vi "04-ClusterEscala.vi"() -> ()   [LabVIEW 2020]
panel:
  in  "Tab Control":enum32{"Cluster"}(tab)
  out "Cluster":T1 {"Tank" scale=0.0..500.0; "Gauge" scale=0.0..500.0; "Thermometer" scale=0.0..100.0}
  in  "Cluster 2":T2
  out "x*y":cluster{dbl, dbl, dbl}
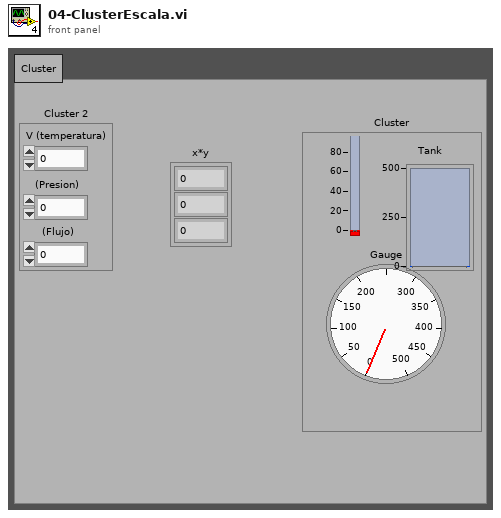
[diagram p1: front panel]
types:
  T1 = cluster{"Thermometer":dbl, "Gauge":dbl, "Tank":dbl}
  T2 = cluster{"V (temperatura)":dbl, "(Presion)":dbl, "(Flujo)":dbl}
  T3 = cluster{"°C/V":i32, "(I/seg)/V":i32, "(N/m^2)/V":i32}
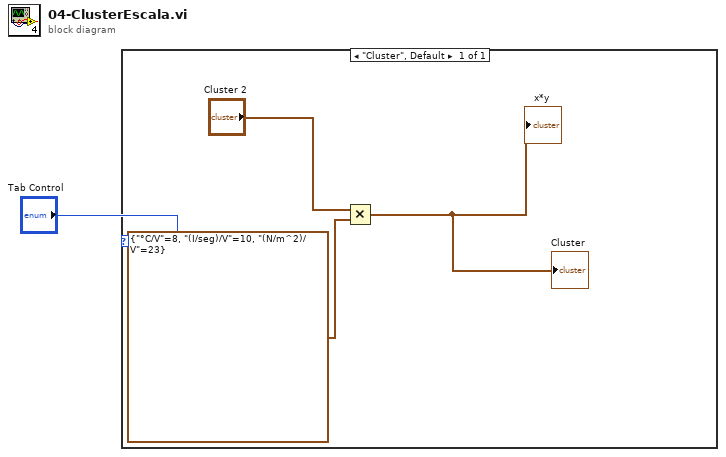
[diagram p0: block diagram]
diagram:
  n1 = case shown="\"Cluster\", Default" "Tab Control" {
    frame "Cluster", Default {
      n2 = Multiply(x="Cluster 2", y=T3 {"°C/V"=8, "(I/seg)/V"=10, "(N/m^2)/V"=23}) -> (x*y=→"x*y" →"Cluster":cluster{dbl, dbl, dbl})
    }
  }
